vi "Initialize Channel Parameter (Discrete).vi"(6 "index":i32, 10 "default value (0)":dbl, 11 "name":string) -> (3 "channel parameter":T1={"name"="", "default value"=0.0, "unit"="", "Parameter"={"start index"=0, "size"=1, "encoding"=enum."BNR", "signed"=FALSE, "scale multiplier"=1.0, "scale offset"=0.0}})   [LabVIEW 2020]
uses:
  VS Channel Definition for Parameter.ctl
  Users/nitest/Desktop/Source_snapshot_20210209/Protocol/Implementations/ARINC429/Parameter Definition.ctl
  Users/nitest/Desktop/Source_snapshot_20210209/Encoding and Decoding/Encoding.ctl
  Users/nitest/Desktop/Source_snapshot_20210209/Encoding and Decoding/Encoding and Decoding.lvlib
  Users/nitest/Desktop/Source_snapshot_20210209/Protocol/Implementations/ARINC429/ARINC 429.lvclass
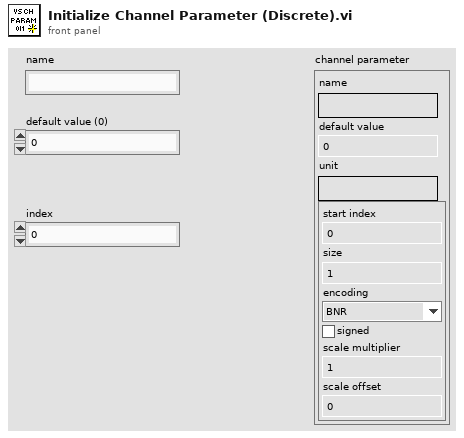
[diagram p1: front panel]
types:
  T1 = typedef "VS Channel Definition for Parameter.ctl" = cluster{"name":string, "default value":dbl, "unit":string, "Parameter":T2}
  T2 = typedef "ARINC 429.lvclass/Parameter Definition.ctl" = cluster{"start index":i32, "size":i32, "encoding":T3, "signed":bool, "scale multiplier":dbl, "scale offset":dbl}
  T3 = typedef "Encoding and Decoding.lvlib/Encoding.ctl" = enum16{"BNR", "BCD", "Discrete"}
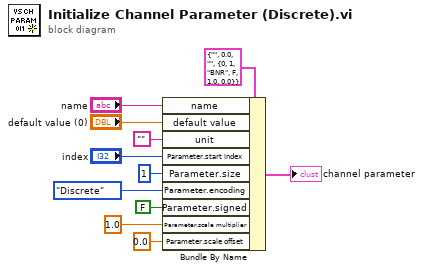
[diagram p0: block diagram]
diagram:
  n1 = Bundle By Name(cluster=T1 {"name"="", "default value"=0.0, "unit"="", "Parameter"={"start index"=0, "size"=1, "encoding"=enum."BNR", "signed"=FALSE, "scale multiplier"=1.0, "scale offset"=0.0}} ("channel parameter"), "name"="name", "default value"="default value (0)", "unit"="", "Parameter.start index"="index", "Parameter.size"=1 ("size"), "Parameter.encoding"=Encoding."Discrete", "Parameter.signed"=FALSE, "Parameter.scale multiplier"=1.0, "Parameter.scale offset"=0.0) -> (→"channel parameter":T1)
